vi "global current shutter.vi"() -> ()   [LabVIEW 2014]
panel:
  out "String":string
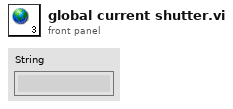
[diagram p1: front panel]
diagram:
